vi "compare target and actual motor positions.vi"(1 "y":dbl, 2 "Target Motor Positions":T1, 3 "Motor Positions Actual":T2) -> (0 "Boolean":bool)   [LabVIEW 2011]
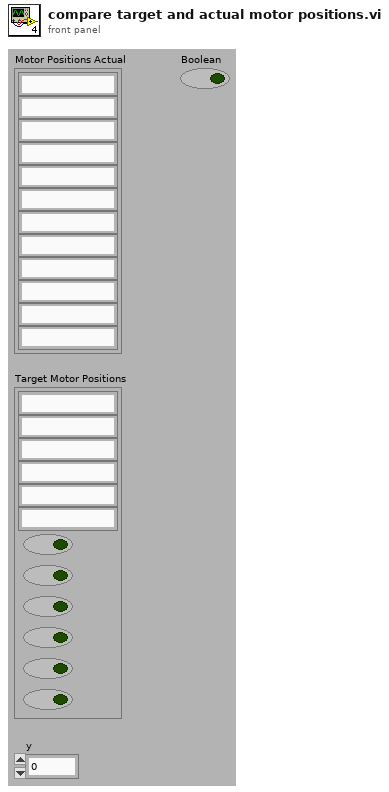
[diagram p1: front panel]
types:
  T1 = cluster{string, string, string, string, string, string, bool, bool, bool, bool, bool, bool}
  T2 = cluster{string, string, string, string, string, string, string, string, string, string, string, string}
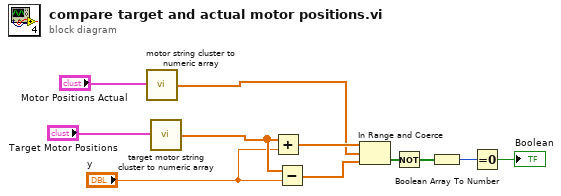
[diagram p0: block diagram]
diagram:
  n1 = call "motor string cluster to numeric array.vi"("Motor Positions Actual"="Motor Positions Actual") -> ("Array"=w2:dbl[])
  n2 = call "target motor string cluster to numeric array.vi"("Target Motor Positions"="Target Motor Positions") -> ("Array"=w5:dbl[])
  n3 = Add(x=w5, y="y") -> (x+y=w3:dbl[])
  n4 = Subtract(x=w5, y="y") -> (x-y=w1:dbl[])
  n5 = In Range and Coerce(upper limit=w3, x=w2, lower limit=w1) -> (In Range?=w8:bool[])  [unwired: 1 out]
  n6 = Not(x=w8) -> (.not. x?=w9:bool[])
  n7 = Boolean Array To Number(Boolean array=w9) -> (number=w10:u32)
  n8 = Equal To 0?(x=w10) -> (x = 0?=→"Boolean":bool)
